vi "Get Universal Timeout.vi"(8 "error in (no error)":errorcluster, 11 "LabVIEWHTTPClient_NET in":refnum<class "HttpClient_NET.lvclass">) -> (0 "error out":errorcluster, 2 "Seconds":dbl, 3 "LabVIEWHTTPClient_NET out":refnum<class "HttpClient_NET.lvclass">)   [LabVIEW 2018, in "HttpClient_NET.lvlib" / "HttpClient_NET.lvclass"]
doc: "<b> </b> <b> </b>\nHttpClient_NET\nJustin Young - Viviota\nCopyright (c) 2021\nLicense: BSD"
uses:
  HttpClient_NET.lvclass
  HttpClient_NET.lvclass/HttpClient_NET.ctl
  Accessors/Read NET_HttpClient.vi
  System.Net.Http
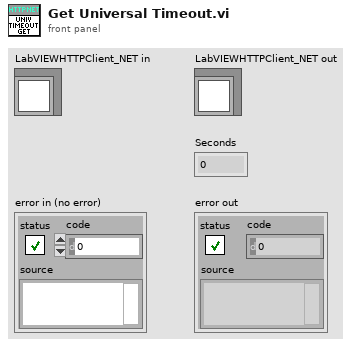
[diagram p1: front panel]
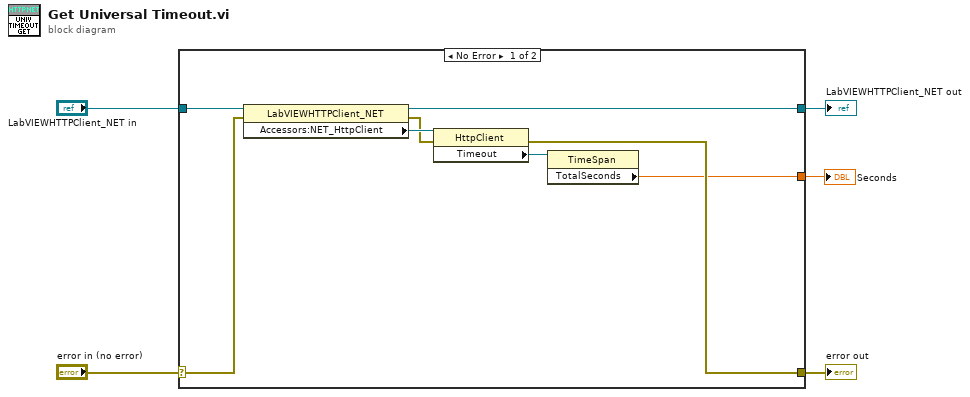
[diagram p0: block diagram]
diagram:
  n1 = case shown="No Error" "error in (no error)" {
    selector: "error in (no error)" -> [w10 w15]
    tunnel: [w8 w15] -> w4
    tunnel: [w12 w14] -> w2
    tunnel: "LabVIEWHTTPClient_NET in" -> [w13 w14]
    tunnel: [w6 _] -> w1
    frame No Error {
      n2 = property class="LabVIEWHTTPClient_NET"(reference=w13, error in=w10) -> (reference out=w12:refnum<class "HttpClient_NET.lvclass">, error out=w9:errorcluster, "Accessors:NET_HttpClient"=w11:refnum<k24>)
      n3 = property class="HttpClient"(reference=w11, error in=w9) -> (error out=w8:errorcluster, "Timeout"=w7:refnum<k24>)  [unwired: 1 out]
      n4 = property class="TimeSpan"(reference=w7) -> ("TotalSeconds"=w6:dbl)  [unwired: 1 in, 2 out]
    }
    frame Error {
    }
  }
  "error out" <- w4
  "LabVIEWHTTPClient_NET out" <- w2
  "Seconds" <- w1
